vi "Configure List Mode Sweep.vi"(0 "VISA resource name":refnum<visa-resource-name>, 1 "Source Mode  (0: Voltage)":u16(ring) items=["Voltage", "Current"], 5 "Start Index(1)":u32=1, 7 "Delay (0)":dbl format="%#_9g", 9 "Count (1)":i32=1, 11 "error in (no error)":errorcluster, 12 "Fail Abort (T:ON)":bool=TRUE, 13 "Buffer Name (defbuffer1)":string="defbuffer1", 14 "Configuration List Name":string) -> (4 "VISA resource name out":refnum<visa-resource-name>, 15 "error out":errorcluster)   [LabVIEW 2021, in "Keithley 2450.lvlib"]
doc: "This sets up a sweep based on a configuration list, which allows you to customize the sweep."
uses:
  <instrlib>/Keithley 2450/Keithley 2450.lvlib
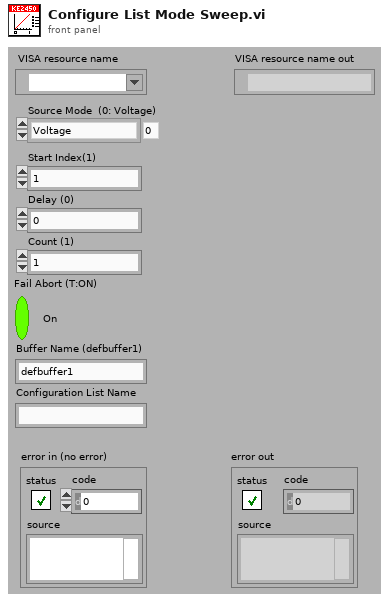
[diagram p1: front panel]
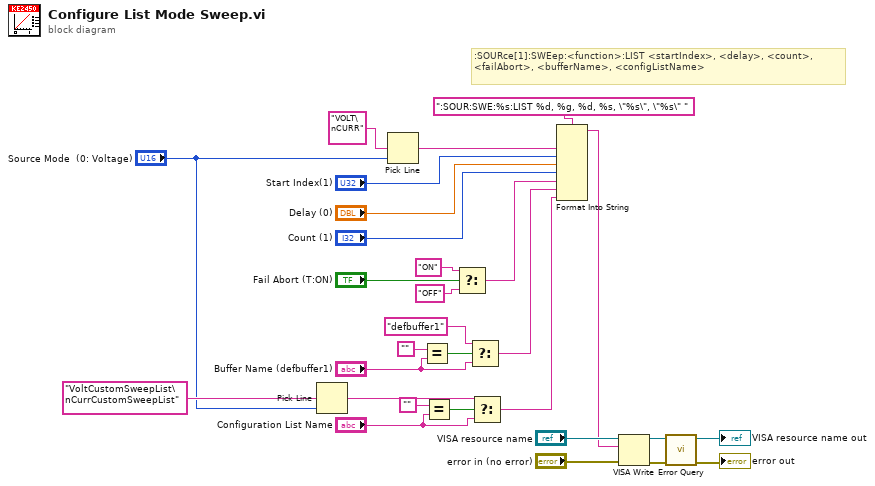
[diagram p0: block diagram]
diagram:
  # ":SOURce[1]:SWEep:<function>:LIST <startIndex>, <delay>, <count>, <failAbort>, <bufferName>, <configListName>"
  n1 = Pick Line(multi-line string="VoltCustomSweepList\nCurrCustomSweepList" ("string (\"\")"), line index="Source Mode  (0: Voltage)") -> (output string=w1:string)  [unwired: 1 out]
  n2 = Pick Line(multi-line string="VOLT\nCURR" ("string (\"\")"), line index="Source Mode  (0: Voltage)") -> (output string=w27:string)  [unwired: 1 out]
  n3 = Equal?(x="", y="Buffer Name (defbuffer1)") -> (x = y?=w15:bool)
  n4 = Equal?(x="", y="Configuration List Name") -> (x = y?=w7:bool)
  n5 = Select(t="ON" ("Buffer Name (defbuffer1)"), s="Fail Abort (T:ON)", f="OFF" ("Buffer Name (defbuffer1)")) -> (s? t:f=w9:string)
  n6 = Select(t="defbuffer1", s=w15, f="Buffer Name (defbuffer1)") -> (s? t:f=w8:string)
  n7 = Select(t=w1, s=w7, f="Configuration List Name") -> (s? t:f=w4:string)
  n8 = Format Into String(format string=":SOUR:SWE:%s:LIST %d, %g, %d, %s, \"%s\", \"%s\" ", w27, "Start Index(1)", "Delay (0)", "Count (1)", w9, w8, w4) -> (resulting string=w19:string)  [unwired: 2 in, 1 out]
  n9 = VISA Write(VISA resource name="VISA resource name", write buffer=w19, error in (no error)="error in (no error)") -> (VISA resource name out=w24:refnum<visa-resource-name>, error out=w23:errorcluster)  [unwired: 1 out]
  n10 = call <instrlib>:"Error Query.vi"("error in (no error)"=w23, "VISA resource name"=w24) -> ("error out"=→"error out":errorcluster, "VISA resource name out"=→"VISA resource name out":refnum<visa-resource-name>)  [unwired: 8 out]
